vi "PC_StateMachine.vi"() -> ()   [LabVIEW 2009]
doc: "Use this template to build a producer/consumer design pattern with events to produce queue items. Use this design pattern instead of the User Interface Event Handler pattern for user interfaces when you want to execute code asynchronously in response to an event without slowing the user interface responsiveness."
panel:
  out "P-State":string="Timeout"
  in  "Cal-3":bool
  in  "Cal-2":bool
  in  "Cal-1":bool
  out "C-State":string
  in  "Calibrate":bool
  in  "stop":bool
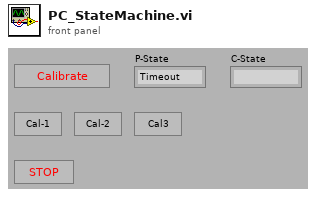
[diagram p1: front panel]
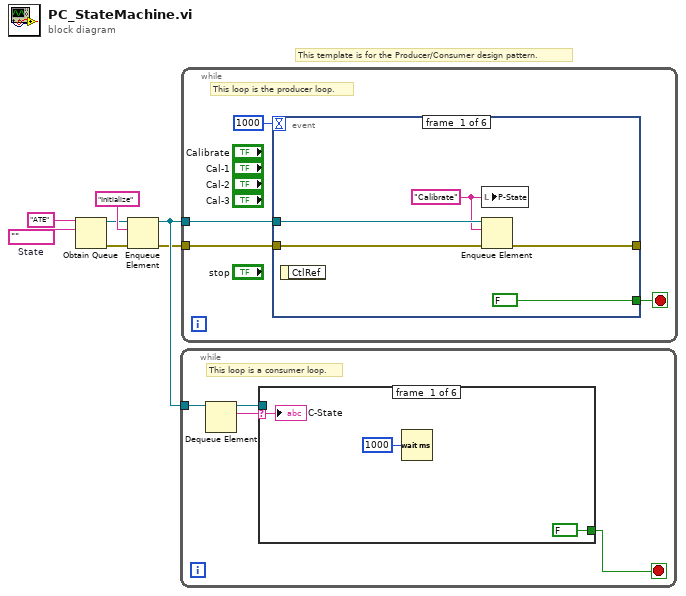
[diagram p0: block diagram]
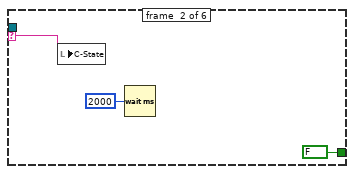
[diagram p2: hidden frame]
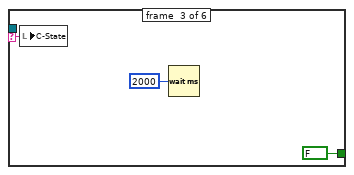
[diagram p3: hidden frame]
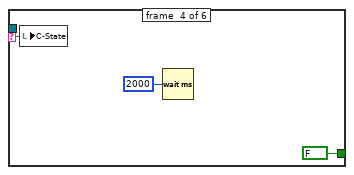
[diagram p4: hidden frame]
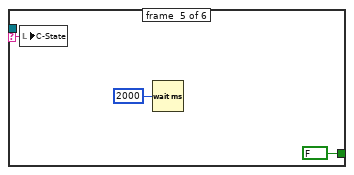
[diagram p5: hidden frame]
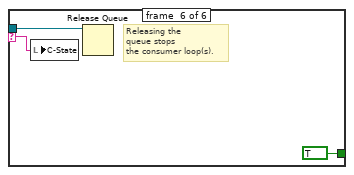
[diagram p6: hidden frame]
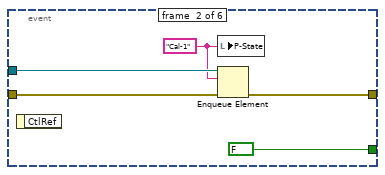
[diagram p7: hidden frame]
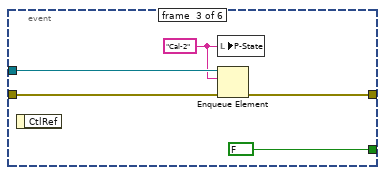
[diagram p8: hidden frame]
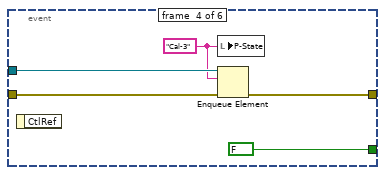
[diagram p9: hidden frame]
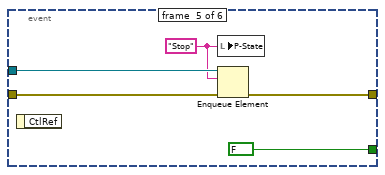
[diagram p10: hidden frame]
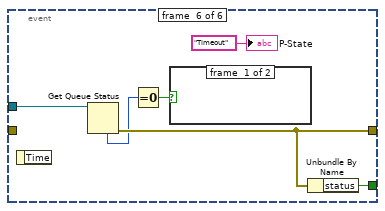
[diagram p11: hidden frame]
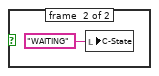
[diagram p12: hidden frame]
diagram:
  w7 = ""  # State
  # "This template is for the Producer/Consumer design pattern."
  n1 = Obtain Queue(name (unnamed)="ATE", element data type=w7) -> (queue out=w4:refnum<queue>, error out=w2:errorcluster)  [unwired: 3 in, 1 out]
  n2 = Enqueue Element(queue=w4, element="Initialize", error in (no error)=w2) -> (queue out=w3:refnum<queue>, error out=w1:errorcluster)  [unwired: 1 in, 1 out]
  n3 = while {
    tunnel: w3 -> [w11]
    stop <- w8 stop-if-true
    # "This loop is a consumer loop."
    n4 = Dequeue Element(queue=w11) -> (queue out=w9:refnum<queue>, element=w10:string)  [unwired: 2 in, 2 out]
    n5 = case shown="\"Cal-2\"" w10 {
      selector: w10 -> [w13 w16 w19 w22 w25 w28]
      tunnel: w9 -> [_ _ _ _ _ w27]
      tunnel: [FALSE FALSE FALSE FALSE FALSE TRUE] -> w8
      frame #0 {
        n6 = Wait (ms)(milliseconds to wait=u32 1000) -> ()  [unwired: 1 out]
        "C-State" <- w13
      }
      frame #1 {
        n7 = local write "C-State"(w16) -> ()
        n8 = Wait (ms)(milliseconds to wait=u32 2000) -> ()  [unwired: 1 out]
      }
      frame #2 {
        n9 = local write "C-State"(w19) -> ()
        n10 = Wait (ms)(milliseconds to wait=u32 2000) -> ()  [unwired: 1 out]
      }
      frame #3 {
        n11 = local write "C-State"(w22) -> ()
        n12 = Wait (ms)(milliseconds to wait=u32 2000) -> ()  [unwired: 1 out]
      }
      frame #4 {
        n13 = local write "C-State"(w25) -> ()
        n14 = Wait (ms)(milliseconds to wait=u32 2000) -> ()  [unwired: 1 out]
      }
      frame #5 {
        # "Releasing the\nqueue stops\nthe consumer loop(s)."
        n15 = local write "C-State"(w28) -> ()
        n16 = Release Queue(queue=w27) -> ()  [unwired: 2 in, 3 out]
      }
    }
  }
  n17 = while {
    tunnel: w3 -> [w33]
    tunnel: w1 -> [w32]
    stop <- w30 stop-if-true
    # "This loop is the producer loop."
    n18 = event shown="[5] Timeout" {
      selector: _ -> [_ _ _ _ _ _]
      dyn-events: _ -> [_ _ _ _ _ _]
      timeout: 1000 -> [_ _ _ _ _ _]
      tunnel: w33 -> [w38 w43 w48 w53 w56 w64]
      tunnel: w32 -> [w37 w42 w47 w52 w58 _]
      tunnel: [w36 w41 w46 w51 w57 w62] -> _
      tunnel: [FALSE FALSE FALSE FALSE FALSE w63] -> w30
      event #0 {
        w34 = "Calibrate" ("element")
        n19 = event-data() -> ()  [unwired: 1 in, 1 out]
        n20 = local write "P-State"(w34) -> ()
        n21 = Enqueue Element(queue=w38, element=w34, error in (no error)=w37) -> (error out=w36:errorcluster)  [unwired: 1 in, 2 out]
      }
      event #1 {
        w39 = "Cal-1" ("element")
        n22 = event-data() -> ()  [unwired: 1 in, 1 out]
        n23 = local write "P-State"(w39) -> ()
        n24 = Enqueue Element(queue=w43, element=w39, error in (no error)=w42) -> (error out=w41:errorcluster)  [unwired: 1 in, 2 out]
      }
      event #2 {
        w44 = "Cal-2" ("element")
        n25 = event-data() -> ()  [unwired: 1 in, 1 out]
        n26 = local write "P-State"(w44) -> ()
        n27 = Enqueue Element(queue=w48, element=w44, error in (no error)=w47) -> (error out=w46:errorcluster)  [unwired: 1 in, 2 out]
      }
      event #3 {
        w49 = "Cal-3" ("element")
        n28 = event-data() -> ()  [unwired: 1 in, 1 out]
        n29 = local write "P-State"(w49) -> ()
        n30 = Enqueue Element(queue=w53, element=w49, error in (no error)=w52) -> (error out=w51:errorcluster)  [unwired: 1 in, 2 out]
      }
      event #4 {
        w54 = "Stop" ("element")
        n31 = event-data() -> ()  [unwired: 1 in, 1 out]
        n32 = local write "P-State"(w54) -> ()
        n33 = Enqueue Element(queue=w56, element=w54, error in (no error)=w58) -> (error out=w57:errorcluster)  [unwired: 1 in, 2 out]
      }
      event #5 {
        n34 = event-data() -> ()  [unwired: 1 in, 1 out]
        n35 = Get Queue Status(queue=w64) -> (error out=w62:errorcluster, # elements in queue=w60:i32)  [unwired: 2 in, 6 out]
        n36 = Equal To 0?(x=w60) -> (x = 0?=w59:bool)
        n37 = case shown="True" w59 {
          frame #0 {
          }
          frame #1 {
            n38 = local write "C-State"("WAITING" ("element")) -> ()
          }
        }
        n39 = Unbundle By Name(w62) -> ("status"=w63:bool)
        "P-State" <- "Timeout" ("element")
      }
    }
  }
